vi "Modified with AO, Multi-Function-Synch AI-Read Dig Chan (1).vi"() -> ()   [LabVIEW 2019]
doc: "I. Description:\nThis example demonstrates how to continuously acquire analog and digital data at the same time, synchronized with one another on the same device.\n\nII. Instructions for Running:\n1. Select the physical channel to correspond to where your analog signal is input on the DAQ device. Also, select the channel to correspond to where your digital signal is input on the DAQ device.\n2. Enter the minimum and maximum voltage ranges.\nNote: For better accuracy try to match the input range to the expected voltage level of the measured signal.\n3. Set the sample rate of the acquisition.\nNote: The rate should be at least twice as fast as the maximum frequency component of the signal being acquired. \nNote: This example requires two DMA channels to run. If your hardware does not support two DMA channels, you need to set the Data Transfer Mechanism property for the Digital Input Task to use \"Interrupts\". The Data Transfer Mechanism property is located in the DAQmx Channel Property hierarchy at:\n\nDAQmx Channel Property Node>>Digital Input>>General Properties>>Advanced>>Data Transfer and Memory>>Data Transfer Mechanism\n\nRefer to your device documentation to determine how many DMA channels are supported for your hardware.\n\nIII. Block Diagram Steps:\n1. Create an analog input voltage channel. Also, create a Digital Input channel.\n2. Set the rate for the sample clockz. Additionally, define the sample modez to be continuous. \n2a. Call the Get Terminal Name with Device Prefix VI. This will take a Task and a terminal and create a properly formatted device + terminal name to use as the source of the digital sample clock.\n3. Call the Start VI to arm the two functions. Make sure the digital input task is armed before the analog input task. This will ensure both will start at the same time.\n4. Read the waveform data in a loop until the user hits the stop button or an error occurs. \n5. Call the Clear VI to Clear the Tasks\n6. Use the popup dialog box to display an error if any.\n\nIV. I/O Connections Overview:\nMake sure your signal input terminals match the Physical Channel I/O controls."
uses:
  <vilib>/Utility/error.llb/DialogType.ctl
  <vilib>/DAQmx/write.llb/DAQmx Write (Analog Wfm 1Chan NSamp).vi
  <vilib>/DAQmx/read.llb/DAQmx Read (Analog Wfm 1Chan NSamp).vi
  <vilib>/DAQmx/read.llb/DAQmx Read (Digital Wfm 1Chan NSamp).vi
  <vilib>/DAQmx/create/channels.llb/DAQmx Create Channel (AI-Voltage-Basic).vi
  <vilib>/DAQmx/configure/timing.llb/DAQmx Timing (Sample Clock).vi
  <vilib>/DAQmx/create/channels.llb/DAQmx Create Channel (DI-Digital Input).vi
  <vilib>/DAQmx/create/channels.llb/DAQmx Create Channel (AO-Voltage-Basic).vi
  <vilib>/DAQmx/miscellaneous.llb/DAQmx Fill In Error Info.vi
  <vilib>/DAQmx/configure/trigger.llb/DAQmx Start Trigger (Digital Edge).vi
  <vilib>/measure/NI_MABase.lvlib
panel:
  in  "Trigger Source":tag="/Dev1/PFI0"
  out "Sample Clock Source":tag="/Dev1/ai/SampleClock"
  in  "Amplitude":dbl=1.0 format="%0.2p"
  in  "Signal Type":T1(ring)
  in  "minimum output value":dbl=-10.0 caption="Output Minimum Value" format="%0.2f"
  in  "maximum output value":dbl=10.0 caption="Output Maximum Value" format="%0.2f"
  in  "physical channels":tag="Dev1/ao0" caption="Output Physical Channels"
  out "Digital Measurement":digitalwaveform(graph)={"t0"=timestamp(3736156304.6237516 s since 1904-01-01), "dt"=9.999999999999999e-05, "Y"={"transitions"=[], "data"=array1000x8[8000 elements]}, "attributes"=variant("NI_ChannelName"=variant(string "Dev1/port0"), "NI_LineNames"=variant(string "Dev1/port0/line7,Dev1/port0/line6,Dev1/port0/line5,Dev1/port0/line4,Dev1/port0/line3,Dev1/port0/line2,Dev1/port0/line1,Dev1/port0/line0"))}
  in  "Digital Input Physical Channel":tag="Dev1/port0"
  in  "Samples to Read":i32=1000
  in  "Maximum Input Value":dbl=10.0 caption="Input Maximum Value" format="%0.2f"
  in  "Minimum Input Value":dbl=-10.0 caption="Input Minimum Value" format="%0.2f"
  in  "Analog Input Physical Channel":tag="Dev1/ai0"
  in  "Rate":dbl=10000.0 caption="Input Rate" format="%0.2f"
  in  "stop":bool
  out "Measurement":waveform(dbl)(graph)={"t0"=timestamp(3736156304.6679516 s since 1904-01-01), "dt"=9.999999999999999e-05, "Y"=array[1000 elements], "attributes"=variant("NI_ChannelName"=variant(string "Dev1/ai0"), "NI_UnitDescription"=variant(string "Volts"))} caption="Analog Measurement"
  # "For instructions, select Help>>Show Context Help"
  # "Channel Parameters"
  # "Analog Output Parameters"
  # "Timing Parameters"
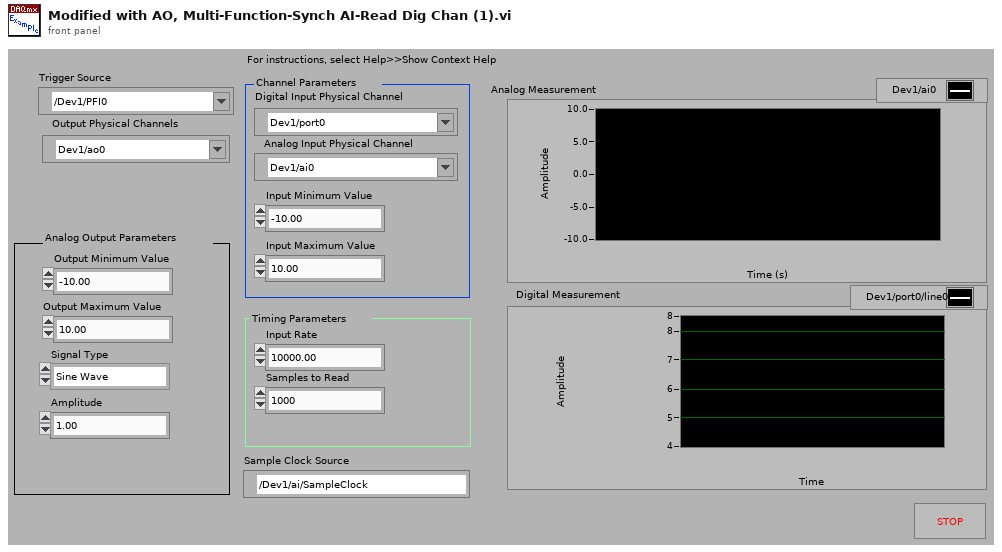
[diagram p1: front panel]
types:
  T1 = enum16{"Sine Wave", "Triangle Wave", "Square Wave", "Sawtooth Wave"}
  T2 = typedef "DialogType.ctl" = u16
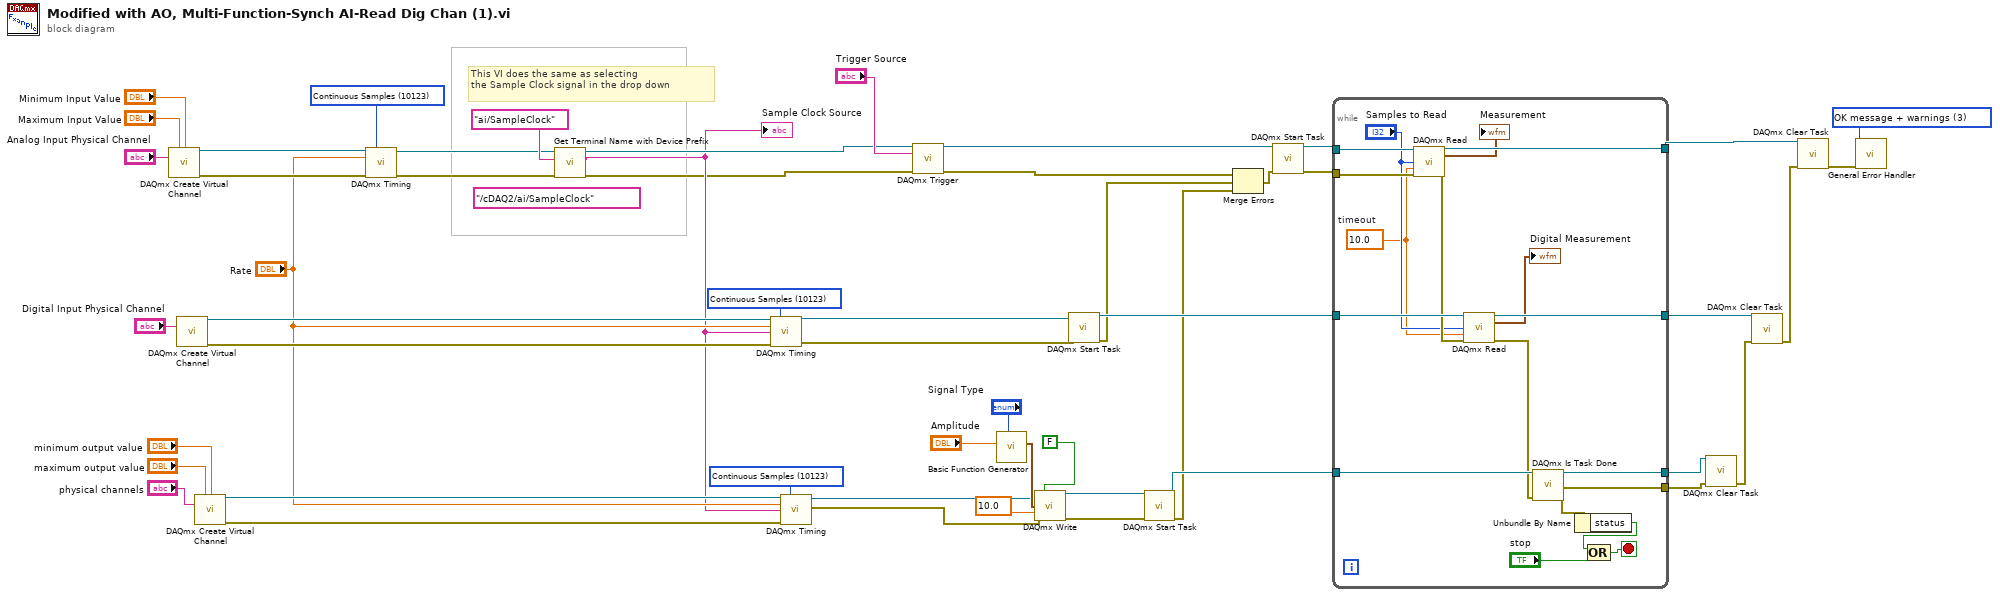
[diagram p0: block diagram]
diagram:
  (unwired) tag "/cDAQ2/ai/SampleClock" ("Terminal Name with Device Prefix")
  w27 = 10123 items=["Finite Samples"=10178, "Continuous Samples"=10123] ("sample mode")
  w42 = T2 3 items=["no dialog", "OK message", "continue or stop message", "OK message + warnings", "continue/stop + warnings"] ("type of dialog (OK msg:1)")
  w46 = 10123 items=["Finite Samples"=10178, "Continuous Samples"=10123] ("sample mode")
  w49 = 10123 items=["Finite Samples"=10178, "Continuous Samples"=10123] ("sample mode")
  # "This VI does the same as selecting\nthe Sample Clock signal in the drop down"
  n1 = call-poly <vilib>:"DAQmx Create Virtual Channel.vi"("maximum value"="Maximum Input Value", "minimum value"="Minimum Input Value", "physical channels"="Analog Input Physical Channel") -> ("task out"=w47:refnum<k21>, "error out"=w48:errorcluster)  [unwired: 11 in]
  n2 = call-poly <vilib>:"DAQmx Create Virtual Channel.vi"("lines"="Digital Input Physical Channel") -> ("task out"=w45:refnum<k21>, "error out"=w44:errorcluster)  [unwired: 13 in]
  n3 = call-poly <vilib>:"DAQmx Create Virtual Channel.vi"("maximum value"="maximum output value", "minimum value"="minimum output value", "physical channels"="physical channels") -> ("task out"=w26:refnum<k21>, "error out"=w25:errorcluster)  [unwired: 11 in]
  n4 = call-poly <vilib>:"DAQmx Timing.vi"("task/channels in"=w47, "sample mode"=w49, "rate"="Rate", "error in"=w48) -> ("task out"=w3:refnum<k21>, "error out"=w4:errorcluster)  [unwired: 10 in]
  n5 = call "Get Terminal Name with Device Prefix.vi"("error in (no error)"=w4, "Local Terminal Name"="ai/SampleClock", "task/channels in"=w3) -> ("error out"=w1:errorcluster, "Terminal Name with Device Prefix"=w2:tag, "task out"=w5:refnum<k21>)  [unwired: 6 in]
  "Sample Clock Source" <- w2
  n6 = call-poly <vilib>:"DAQmx Timing.vi"("task/channels in"=w45, "sample mode"=w46, "rate"="Rate", "source"=w2, "error in"=w44) -> ("task out"=w33:refnum<k21>, "error out"=w32:errorcluster)  [unwired: 9 in]
  n7 = call-poly <vilib>:"DAQmx Timing.vi"("task/channels in"=w26, "sample mode"=w27, "rate"="Rate", "source"=w2, "error in"=w25) -> ("task out"=w9:refnum<k21>, "error out"=w8:errorcluster)  [unwired: 9 in]
  n8 = call-poly <vilib>:"DAQmx Trigger.vi"("task/channels in"=w5, "source"="Trigger Source", "error in"=w1) -> ("task out"=w12:refnum<k21>, "error out"=w13:errorcluster)  [unwired: 11 in]
  n9 = call <vilib>:"Basic Function Generator.vi"("signal type"="Signal Type", "amplitude"="Amplitude") -> ("signal out"=w21:waveform(dbl))  [unwired: 7 in, 2 out]
  n10 = call-poly <vilib>:"DAQmx Write.vi"("task/channels in"=w9, "auto start"=FALSE, "data"=w21, "timeout"=10.0 ("Wirite Timeout"), "error in"=w8) -> ("task out"=w23:refnum<k21>, "error out"=w22:errorcluster)  [unwired: 8 in, 1 out]
  n11 = call <vilib>:"DAQmx Start Task.vi"("task/channels in"=w33, "error in"=w32) -> ("task out"=w43:refnum<k21>, "error out"=w39:errorcluster)  [unwired: 12 in]
  n12 = call <vilib>:"DAQmx Start Task.vi"("task/channels in"=w23, "error in"=w22) -> ("task out"=w18:refnum<k21>, "error out"=w16:errorcluster)  [unwired: 12 in]
  n13 = Merge Errors(w13, w39, w16) -> (w38:errorcluster)
  n14 = call <vilib>:"DAQmx Start Task.vi"("task/channels in"=w12, "error in"=w38) -> ("task out"=w40:refnum<k21>, "error out"=w37:errorcluster)  [unwired: 12 in]
  n15 = while {
    tunnel: [w69] -> w50
    tunnel: w43 -> [w65]
    tunnel: w40 -> [w67]
    tunnel: w37 -> [w66]
    tunnel: [w63] -> w31
    tunnel: [w53] -> w15
    tunnel: w18 -> [w59]
    tunnel: [w58] -> w17
    stop <- w55 stop-if-true
    w61 = 10.0  # timeout
    n16 = call-poly <vilib>:"DAQmx Read.vi"("task/channels in"=w67, "number of samples per channel"="Samples to Read", "timeout"=w61, "error in"=w66) -> ("task out"=w69:refnum<k21>, "data"=→"Measurement":waveform(dbl), "error out"=w64:errorcluster)  [unwired: 9 in]
    n17 = call-poly <vilib>:"DAQmx Read.vi"("task/channels in"=w65, "number of samples per channel"="Samples to Read", "timeout"=w61, "error in"=w64) -> ("task out"=w63:refnum<k21>, "data"=→"Digital Measurement":digitalwaveform, "error out"=w54:errorcluster)  [unwired: 9 in]
    n18 = call <vilib>:"DAQmx Is Task Done.vi"("task/channels in"=w59, "error in"=w54) -> ("task out"=w58:refnum<k21>, "error out"=w53:errorcluster)  [unwired: 11 in, 1 out]
    n19 = Unbundle By Name(w53) -> ("status"=w56:bool)
    n20 = Compound Arithmetic op=OR(w56, "stop") -> (w55:bool)
  }
  n21 = call <vilib>:"DAQmx Clear Task.vi"("task in"=w17, "error in"=w15) -> ("error out"=w14:errorcluster)  [unwired: 13 in]
  n22 = call <vilib>:"DAQmx Clear Task.vi"("task in"=w31, "error in"=w14) -> ("error out"=w36:errorcluster)  [unwired: 13 in]
  n23 = call <vilib>:"DAQmx Clear Task.vi"("task in"=w50, "error in"=w36) -> ("error out"=w35:errorcluster)  [unwired: 13 in]
  n24 = call <vilib>:"General Error Handler.vi"("type of dialog (OK msg:1)"=w42, "error in (no error)"=w35) -> ()  [unwired: 9 in, 5 out]
